vi "Solution Traffic Light.vi"() -> ()   [LabVIEW 2019]
uses:
  Traffic Light States.ctl
panel:
  in  "stop":bool
  out "Red Light":bool
  out "Yellow Light":bool
  out "Green Light":bool
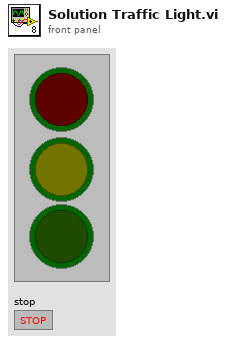
[diagram p1: front panel]
types:
  T1 = typedef "Traffic Light States.ctl" = enum16{"Green", "Yellow", "Red"}
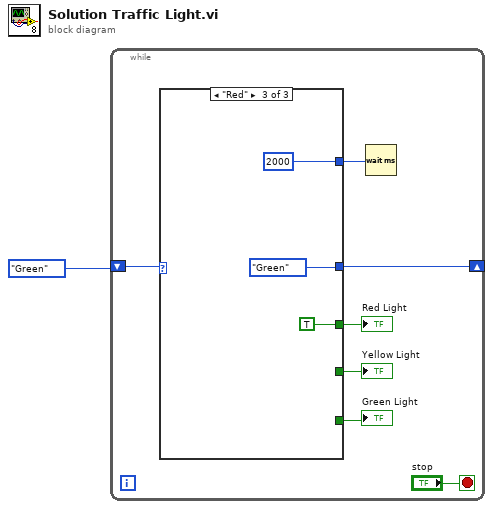
[diagram p0: block diagram]
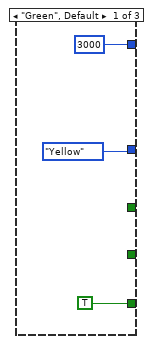
[diagram p2: hidden frame]
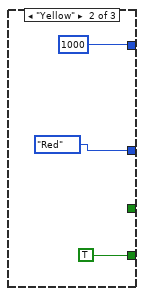
[diagram p3: hidden frame]
diagram:
  n1 = while {
    shift-right: [w7] -> _
    shift-left: Traffic_Light_States."Green" -> [w8]
    stop <- "stop" stop-if-true
    n2 = case shown="\"Red\"" w8 {
      tunnel: [Traffic_Light_States."Yellow" Traffic_Light_States."Red" Traffic_Light_States."Green"] -> w7
      tunnel: [_ _ TRUE] -> w6
      tunnel: [_ TRUE _] -> w5
      tunnel: [TRUE _ _] -> w4
      tunnel: [3000 1000 2000] -> w3
      frame "Green", Default {
      }
      frame "Yellow" {
      }
      frame "Red" {
      }
    }
    "Green Light" <- w4
    "Yellow Light" <- w5
    "Red Light" <- w6
    n3 = Wait (ms)(milliseconds to wait=w3) -> ()  [unwired: 1 out]
  }
